vi "Seriell schreiben.vi"(8 "error in":errorcluster caption="error out", 10 "String":string, 11 "VISA resource name":refnum<visa-resource-name>) -> (0 "error out 2":errorcluster caption="error out", 2 "Verknüpfter String":string, 3 "VISA resource name":refnum<visa-resource-name>)   [LabVIEW 2020, in "AK-Schnittstelle.lvlib" / "AK Seriell.lvlib"]
uses:
  AK Seriell/AK Seriell.lvlib
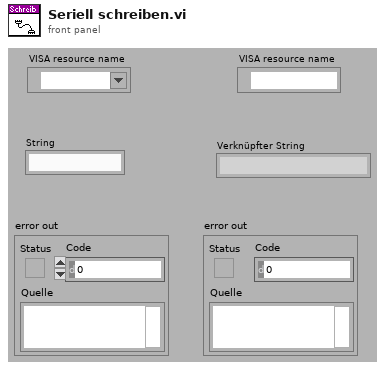
[diagram p1: front panel]
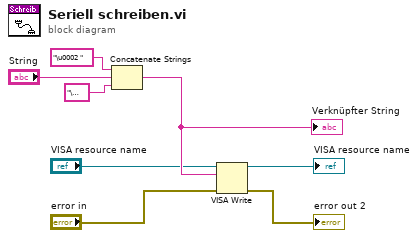
[diagram p0: block diagram]
diagram:
  n1 = Concatenate Strings("\u0002 " ("String"), "String", "\u0003" ("String")) -> (w8:string)
  "Verknüpfter String" <- w8
  n2 = VISA Write(VISA resource name="VISA resource name", write buffer=w8, error in (no error)="error in") -> (VISA resource name out=→"VISA resource name":refnum<visa-resource-name>, error out=→"error out 2":errorcluster)  [unwired: 1 out]
